vi "Flock_Revision_Process.vi"(9 "httpRequestID":u32, 11 "Resource":T1(ring)) -> (0 "source":string, 1 "code":i32, 2 "status":bool, 3 "Response":string)   [LabVIEW 2013, in "FA_RevisionResource.lvlib"]
uses:
  FA_RevisionResource.lvlib
  Shared Code/AMC/VI Source/LocalProcessMessaging/Flock_Shared_LocalProcessMessaging.lvlib
  FA_AgentConfig API/source/VI Source/FA_AgentConfig.lvlib
  Shared Code/AMC/VI Source/CentralProcessMessaging/Flock_Shared_CentralProcessMessaging.lvlib
  Shared Code/AMC/VI Source/Error Handling/Flock_ErrorHandling.lvlib
  <vilib>/wsapi/NI_WebServices.lvlib
  FA_LocalStore API/source/VI Source/FA_LocalStore.lvlib
  FA_LocalStore API/source/VI Source/FA_LSSpecialTypes.ctl
  Central Process/StateValue.ctl
  Central Process/FA_Central Process.lvlib
panel:
  in  "Dev":bool
  out "error out":errorcluster
  in  "Process":string="Revision"
  # "Since this will be a web method, we need to define the process queue name at edit time.\nThis web method VI will be started on it own when called externally."
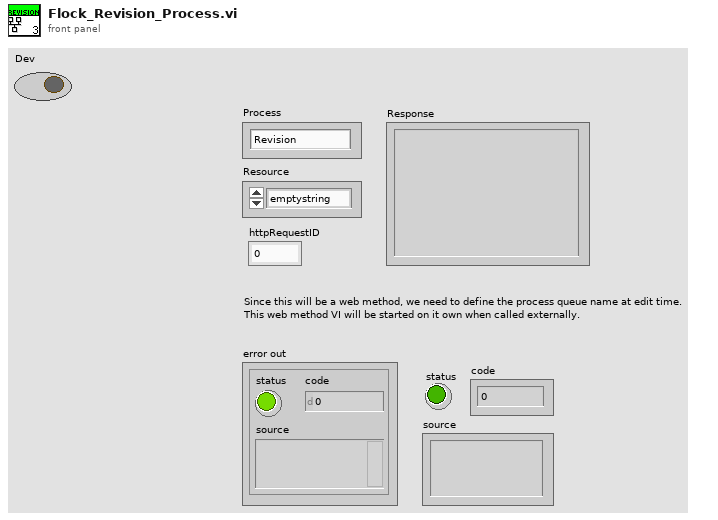
[diagram p1: front panel]
types:
  T1 = enum16{"emptystring", "revision", "deviceconfig", "checkupdateavailable", "forceupdate"}
  T2 = typedef "Flock_Shared_Messaging.lvlib/ProcessList.ctl" = string
  T3 = typedef "FA_LocalStore.lvlib/FA_LSSpecialTypes.ctl" = string
  T4 = typedef "FA_Central Process.lvlib/StateValue.ctl" = enum16{"Available", "Working"}
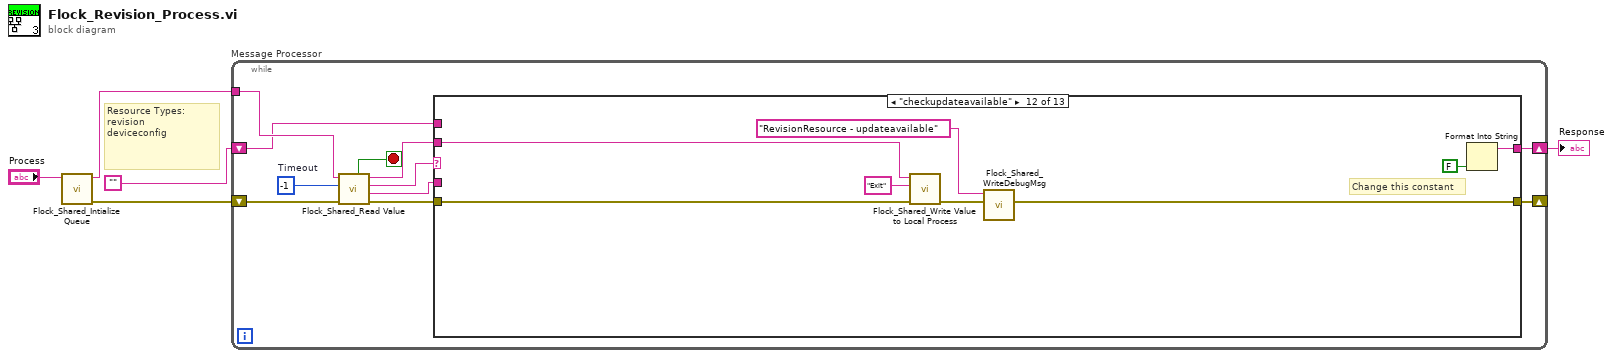
[diagram p0: block diagram]
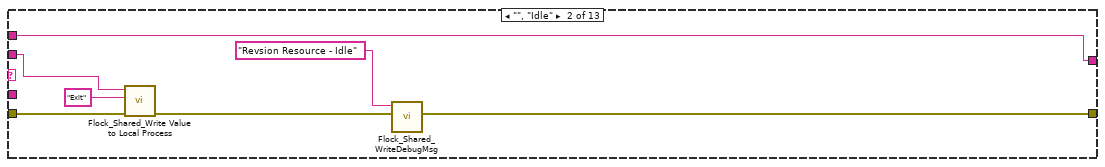
[diagram p3: hidden frame]
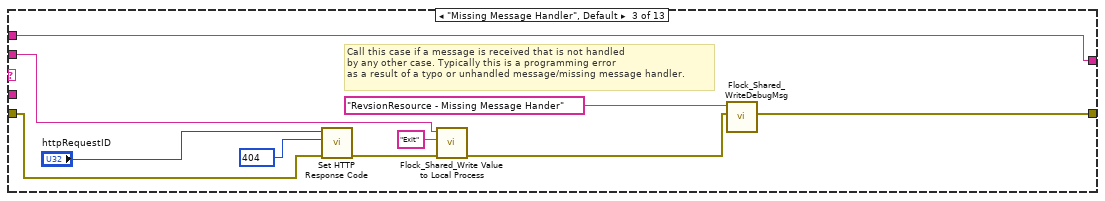
[diagram p4: hidden frame]
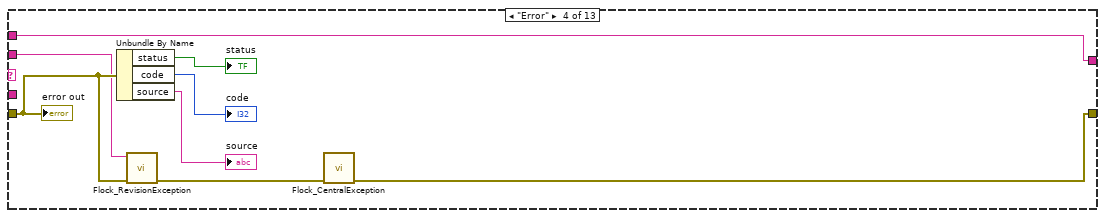
[diagram p5: hidden frame]
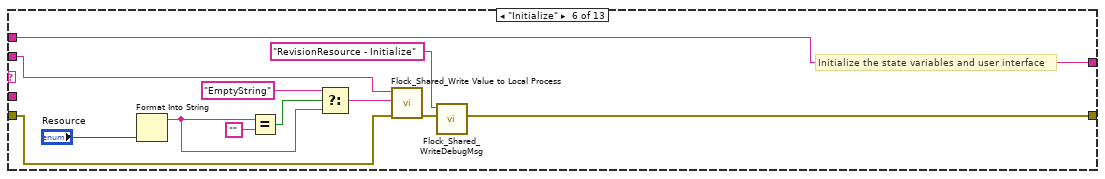
[diagram p7: hidden frame]
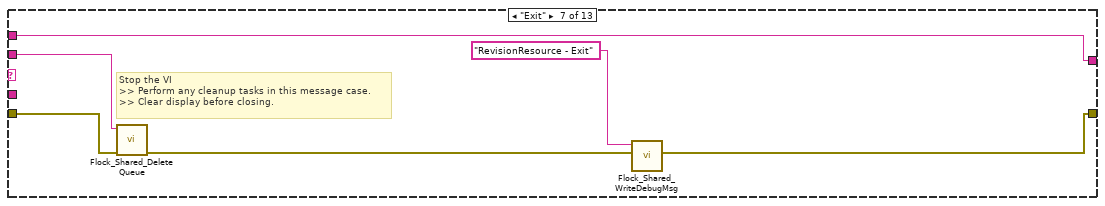
[diagram p8: hidden frame]
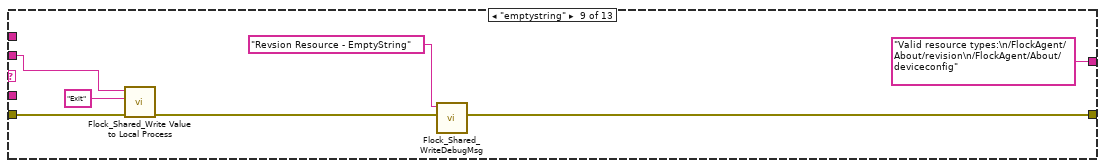
[diagram p10: hidden frame]
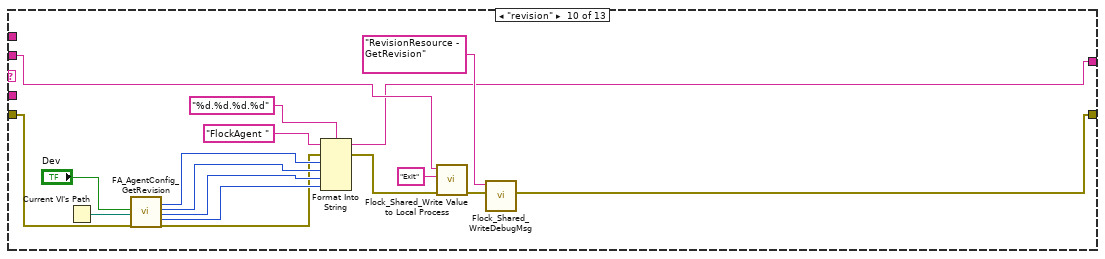
[diagram p11: hidden frame]
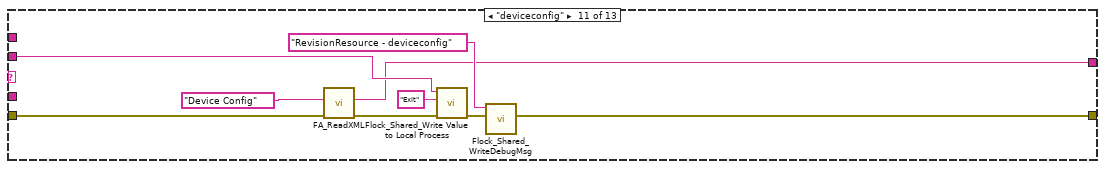
[diagram p12: hidden frame]
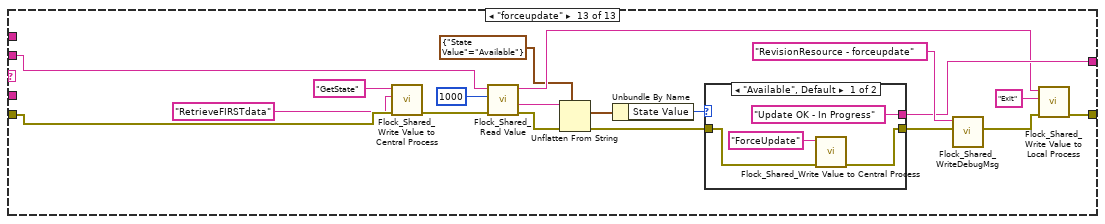
[diagram p13: hidden frame]
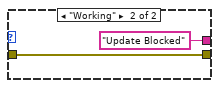
[diagram p14: hidden frame]
diagram:
  # "Resource Types:\nrevision\ndeviceconfig"
  n1 = call "Flock_Shared_Intialize Queue.vi"("Enum"="Process") -> ("error out"=w4:errorcluster, "Process Name"=w3:T2)  [unwired: 9 in]
  n2 = while "Message Processor" {
    shift-left: w4 -> [w14]
    shift-right: [w16] -> _
    tunnel: w3 -> [w9]
    shift-right: [w7] -> w1
    shift-left: "" -> [w6]
    stop <- w10 stop-if-true
    w15 = -1  # Timeout
    n3 = call "Flock_Shared_Read Value.vi"("error in (no error)"=w14, "timeout (1ms)"=w15, "Process"=w9) -> ("error out"=w13:errorcluster, "Message Value"=w11:string, "Message Name"=w12:string, "Process"=w8:T2, "Exit Process"=w10:bool)  [unwired: 4 in]
    n4 = case shown="\"checkupdateavailable\"" w12 {
      tunnel: [w18 w25 w26 w38 w45 w54 w60 w65 w72 w79 w95 w106 w115] -> w16
      tunnel: w13 -> [w18 w21 w28 w40 w45 w56 w63 w65 w68 w74 w91 w99 w122]
      tunnel: w11 -> [_ _ _ _ _ _ _ _ _ _ _ _ _]
      tunnel: w8 -> [_ w23 w31 w37 _ w57 w62 _ w70 w86 w98 w102 w118]
      tunnel: [w17 w19 w29 w36 w44 w48 w58 w64 "Valid resource types:\n/FlockAgent/About/revision\n/FlockAgent/About/deviceconfig" w77 w93 w104 w123] -> w7
      tunnel: w6 -> [w17 w19 w29 w36 w44 w48 w58 w64 _ _ _ _ _]
      frame "---------- Framework Operations ----------" {
        # "Dummy case to add a seperator in the Case Structure menu"
      }
      frame "", "Idle" {
        n5 = call "Flock_Shared_Write Value to Local Process.vi"("error in (no error)"=w21, "Message Name"="Exit", "Process List"=w23) -> ("error out"=w20:errorcluster)  [unwired: 8 in]
        n6 = call "Flock_Shared_WriteDebugMsg.vi"("error in (no error)"=w20, "Current Message Case"="Revsion Resource - Idle" ("Message Value")) -> ("error out"=w25:errorcluster)  [unwired: 9 in]
      }
      frame "Missing Message Handler", Default {
        w33 = 404 items=["100"=100, "101"=101, "200"=200, "201"=201, "202"=202, "203"=203, "204"=204, "205"=205, "206"=206, "300"=300, "301"=301, "302"=302, "303"=303, "304"=304, "305"=305, "306"=306, "307"=307, "400"=400, "401"=401, "402"=402, "403"=403, "404"=404, "405"=405, "406"=406, "407"=407, "408"=408, "409"=409, "410"=410, "411"=411, "412"=412, "413"=413, "414"=414, "415"=415, "416"=416, "417"=417, "500"=500, "501"=501, "502"=502, "503"=503, "504"=504, "505"=505] ("response code (200)")
        # "Call this case if a message is received that is not handled \nby any other case. Typically this is a programming error\nas a result of a typo or unhandled message/missing message handler."
        n7 = call <vilib>:"Set HTTP Response Code.vi"("error in (no error)"=w28, "response code (200)"=w33, "httpRequestID"="httpRequestID") -> ("error out"=w32:errorcluster)  [unwired: 7 in, 1 out]
        n8 = call "Flock_Shared_Write Value to Local Process.vi"("error in (no error)"=w32, "Message Name"="Exit", "Process List"=w31) -> ("error out"=w27:errorcluster)  [unwired: 8 in]
        n9 = call "Flock_Shared_WriteDebugMsg.vi"("error in (no error)"=w27, "Current Message Case"="RevsionResource - Missing Message Hander" ("message")) -> ("error out"=w26:errorcluster)  [unwired: 9 in]
      }
      frame "Error" {
        n10 = Unbundle By Name(w40) -> ("status"=→"status":bool, "code"=→"code":i32, "source"=→"source":string)
        n11 = call "Flock_RevisionException.vi"("Error In"=w40, "Process List"=w37) -> ("Error Out"=w39:errorcluster)  [unwired: 9 in]
        n12 = call "Flock_CentralException.vi"("Error In"=w39) -> ("Error Out"=w38:errorcluster)  [unwired: 10 in]
        "error out" <- w40
      }
      frame "---------- Generic Operations ----------" {
        # "Dummy case to add a seperator in the Case Structure menu"
      }
      frame "Initialize" {
        # "Initialize the state variables and user interface"
        n13 = Format Into String("Resource") -> (resulting string=w47:string)  [unwired: 3 in, 1 out]
        n14 = Equal?(x=w47, y="") -> (x = y?=w51:bool)
        n15 = Select(t="EmptyString", s=w51, f=w47) -> (s? t:f=w49:string)
        n16 = call "Flock_Shared_Write Value to Local Process.vi"("error in (no error)"=w56, "Message Name"=w49, "Process List"=w57) -> ("error out"=w55:errorcluster)  [unwired: 8 in]
        n17 = call "Flock_Shared_WriteDebugMsg.vi"("error in (no error)"=w55, "Current Message Case"="RevisionResource - Initialize") -> ("error out"=w54:errorcluster)  [unwired: 9 in]
      }
      frame "Exit" {
        # "Stop the VI\n>> Perform any cleanup tasks in this message case.\n>> Clear display before closing."
        n18 = call "Flock_Shared_Delete Queue.vi"("Error In"=w63, "Process Name"=w62) -> ("Error Out"=w61:errorcluster)  [unwired: 9 in]
        n19 = call "Flock_Shared_WriteDebugMsg.vi"("error in (no error)"=w61, "Current Message Case"="RevisionResource - Exit") -> ("error out"=w60:errorcluster)  [unwired: 9 in]
      }
      frame "---------- Application Operations ----------" {
        # "Dummy case to add a seperator in the Case Structure menu"
      }
      frame "emptystring" {
        n20 = call "Flock_Shared_Write Value to Local Process.vi"("error in (no error)"=w68, "Message Name"="Exit", "Process List"=w70) -> ("error out"=w67:errorcluster)  [unwired: 8 in]
        n21 = call "Flock_Shared_WriteDebugMsg.vi"("error in (no error)"=w67, "Current Message Case"="Revsion Resource - EmptyString" ("Message Value")) -> ("error out"=w72:errorcluster)  [unwired: 9 in]
      }
      frame "revision" {
        n22 = Current VI's Path() -> (path=w76:path)
        n23 = call "FA_AgentConfig_GetRevision.vi"("Dev"="Dev", "Current VI Path"=w76, "Error In"=w74) -> ("MajorRev"=w84:i32, "MinorRev"=w83:i32, "IterationNum"=w82:i32, "BuildNum"=w81:i32, "Error Out"=w73:errorcluster)  [unwired: 11 in, 1 out]
        n24 = Format Into String(format string="%d.%d.%d.%d", initial string="FlockAgent ", error in=w73, w84, w83, w82, w81) -> (resulting string=w77:string, error out=w87:errorcluster)
        n25 = call "Flock_Shared_Write Value to Local Process.vi"("error in (no error)"=w87, "Message Name"="Exit", "Process List"=w86) -> ("error out"=w80:errorcluster)  [unwired: 8 in]
        n26 = call "Flock_Shared_WriteDebugMsg.vi"("error in (no error)"=w80, "Current Message Case"="RevisionResource - GetRevision") -> ("error out"=w79:errorcluster)  [unwired: 9 in]
      }
      frame "deviceconfig" {
        n27 = call "FA_ReadXML.vi"("Error In"=w91, "Special Type"=T3 "Device Config") -> ("Error Out"=w92:errorcluster, "XML String"=w93:string)  [unwired: 6 in]
        n28 = call "Flock_Shared_Write Value to Local Process.vi"("error in (no error)"=w92, "Message Name"="Exit", "Process List"=w98) -> ("error out"=w96:errorcluster)  [unwired: 8 in]
        n29 = call "Flock_Shared_WriteDebugMsg.vi"("error in (no error)"=w96, "Current Message Case"="RevisionResource - deviceconfig") -> ("error out"=w95:errorcluster)  [unwired: 9 in]
      }
      frame "checkupdateavailable" {
        # "Change this constant"
        n30 = call "Flock_Shared_Write Value to Local Process.vi"("error in (no error)"=w99, "Message Name"="Exit", "Process List"=w102) -> ("error out"=w103:errorcluster)  [unwired: 8 in]
        n31 = call "Flock_Shared_WriteDebugMsg.vi"("error in (no error)"=w103, "Current Message Case"="RevisionResource - updateavailable") -> ("error out"=w106:errorcluster)  [unwired: 9 in]
        n32 = Format Into String(FALSE ("input 1")) -> (resulting string=w104:string)  [unwired: 3 in, 1 out]
      }
      frame "forceupdate" {
        n33 = call "Flock_Shared_Write Value to Central Process.vi"("error in (no error)"=w122, "Message Value"="RetrieveFIRSTdata", "Message Name"="GetState") -> ("error out"=w119:errorcluster)  [unwired: 8 in]
        n34 = call "Flock_Shared_Read Value.vi"("error in (no error)"=w119, "timeout (1ms)"=1000, "Process"=w118) -> ("error out"=w108:errorcluster, "Message Value"=w111:string, "Process"=w114:T2)  [unwired: 4 in, 2 out]
        n35 = Unflatten From String(type=cluster{"State Value":T4} {"State Value"=enum."Available"} ("StateInformation"), binary string=w111, error in (no error)=w108) -> (value=w110:cluster{"State Value":T4}, error out=w107:errorcluster)  [unwired: 2 in, 1 out]
        n36 = Unbundle By Name(w110) -> ("State Value"=w109:T4)
        n37 = case shown="\"Available\", Default" w109 {
          tunnel: [w127 w130] -> w124
          tunnel: ["Update OK - In Progress" ("XML String") "Update Blocked" ("XML String")] -> w123
          tunnel: w107 -> [w126 w130]
          frame "Available", Default {
            n38 = call "Flock_Shared_Write Value to Central Process.vi"("error in (no error)"=w126, "Message Name"="ForceUpdate") -> ("error out"=w127:errorcluster)  [unwired: 9 in]
          }
          frame "Working" {
          }
        }
        n39 = call "Flock_Shared_WriteDebugMsg.vi"("error in (no error)"=w124, "Current Message Case"="RevisionResource - forceupdate") -> ("error out"=w116:errorcluster)  [unwired: 9 in]
        n40 = call "Flock_Shared_Write Value to Local Process.vi"("error in (no error)"=w116, "Message Name"="Exit", "Process List"=w114) -> ("error out"=w115:errorcluster)  [unwired: 8 in]
      }
    }
  }
  "Response" <- w1
